vi "Optionen_2_Text.vi"(8 "error in (no error)":errorcluster caption="Fehler (Eingang, kein Fehler)", 9 "Abschnitt":string, 10 "Wartungsintervall:":sgl, 11 "Optionen":T1) -> (0 "error out":errorcluster caption="Fehler (Ausgang)", 3 "Array":string[](array[string]))   [LabVIEW 2020, in "System Einstellungen V2.lvlib"]
uses:
  System Einstellungen V2.lvlib
  Optionen.ctl
  <vilib>/Utility/Data Type/NI_Data Type.lvlib
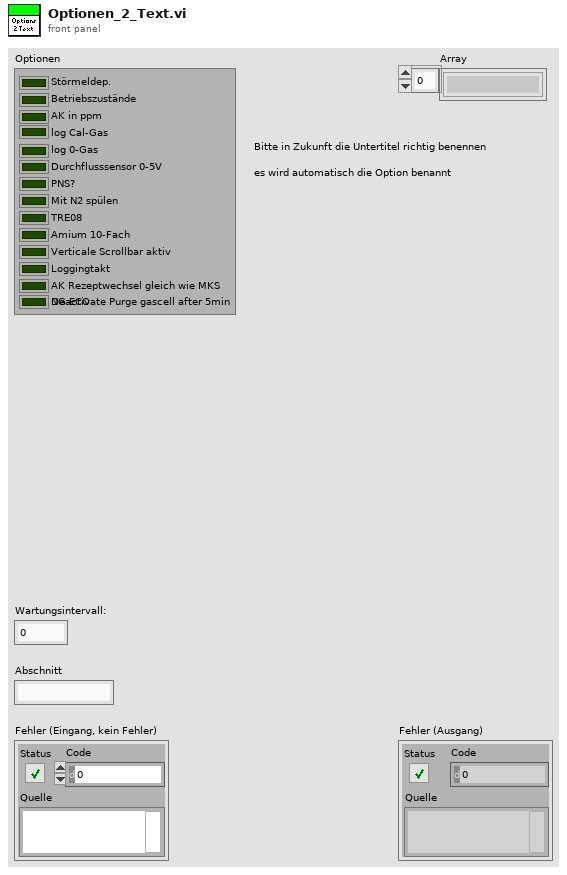
[diagram p1: front panel]
types:
  T1 = typedef "System Einstellungen V2.lvlib/Optionen.ctl" = cluster{"Störmeldep.":bool, "Betriebszustände":bool, "AK in ppm":bool, "log Cal-Gas":bool, "log 0-Gas":bool, "Durchflusssensor 0-5V":bool, "PNS?":bool, "Mit N2 spülen":bool, "TRE08":bool, "Amium 10-Fach":bool, "Verticale Scrollbar aktiv":bool, "Loggingtakt":bool, "AK Rezeptwechsel gleich wie MKS":bool, "NG ECO":bool}
  T2 = typedef "NI_Data Type.lvlib/Data Type.ctl" = enum8{"Invalid Type", "Void", "I8", "I16", "I32", "I64", "U8", "U16", "U32", "U64", "Single Float", "Double Float", "Extended Float", "Single Complex", "Double Complex", "Extended Complex", "Enum U8", "Enum U16", "Enum U32", "Enum U64", "Single Float With Unit", "Double Float With Unit", "Extended Float With Unit", "Single Complex with Unit", "Double Complex with Unit", "Extended Complex with Unit", "Boolean", "String", "Path", "Picture", "Tag", "Array", "Cluster", "Variant", "LV Variant", "Waveform", "Timestamp", "Digital Waveform", "Digital Data", "ExpressData", "Refnum", "External Data", "VI", "Poly VI", "LabVIEW Class Instance", "Fixed Point", "Set Collection", "Map Collection"}
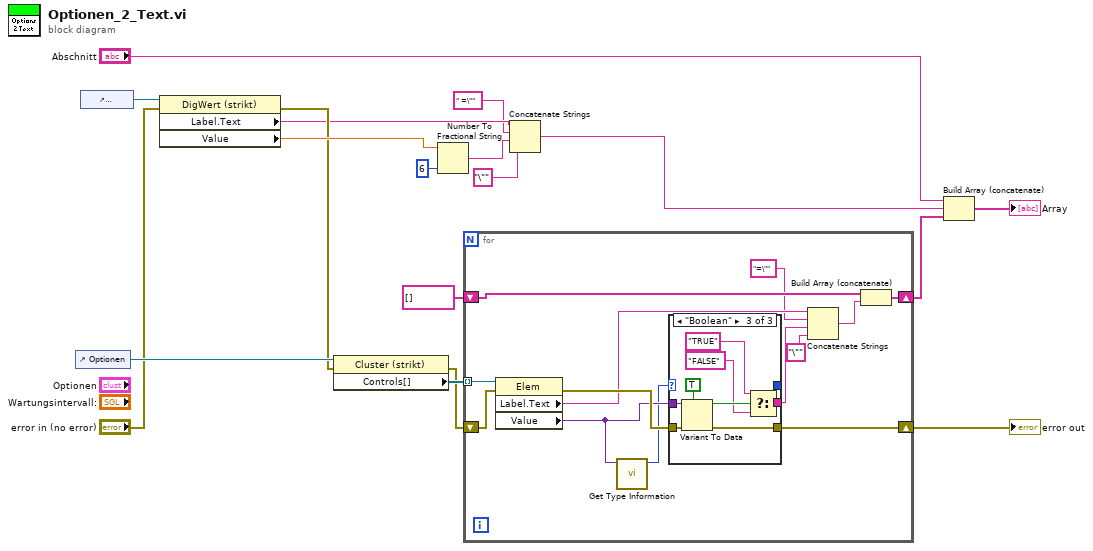
[diagram p0: block diagram]
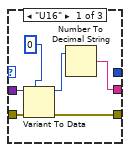
[diagram p2: hidden frame]
diagram:
  n1 = control-ref of="Optionen"() -> (w18:refnum<vi>)
  n2 = control-ref of="Wartungsintervall:"() -> (w12:refnum<vi>)
  n3 = property class="DigWert (strikt)"(reference=w12, error in="error in (no error)") -> (error out=w8:errorcluster, "Label.Text"=w4:string, "Value"=w11:sgl)  [unwired: 1 out]
  n4 = property class="Cluster (strikt)"(reference=w18, error in=w8) -> (error out=w16:errorcluster, "Controls[]"=w17:refnum<vi>[])  [unwired: 1 out]
  n5 = Number To Fractional String(number=w11, precision (6)=i16 6 ("Genauigkeit (6)")) -> (F-format string=w2:string)  [unwired: 2 in]
  n6 = for {
    tunnel: w17 -> [w28] mode=indexing
    shift-right: [w30] -> w15
    shift-left: w16 -> [w29]
    shift-right: [w26] -> w13
    shift-left: string[] [] -> [w25]
    n7 = property class="Elem"(reference=w28, error in=w29) -> (error out=w31:errorcluster, "Label.Text"=w24:string, "Value"=w20:variant)  [unwired: 1 out]
    n8 = call <vilib>:"Get Type Information.vi"("variant"=w20) -> ("type"=w19:T2)  [unwired: 6 in, 4 out]
    n9 = case shown="\"Boolean\"" w19 {
      selector: w19 -> [_ w38 _]
      tunnel: w31 -> [w36 w39 w45]
      tunnel: [w35 w39 w44] -> w30
      tunnel: [w32 _ w41] -> w22
      tunnel: w20 -> [w37 _ w40]
      tunnel: [_ w38 _] -> _
      frame "U16" {
        n10 = Variant To Data(error in=w36, type=u16 0, Variant=w37) -> (data=w33:u16, error out=w35:errorcluster)
        n11 = Number To Decimal String(number=w33) -> (decimal integer string=w32:string)  [unwired: 1 in]
      }
      frame "Invalid Type", Default {
      }
      frame "Boolean" {
        n12 = Variant To Data(error in=w45, type=TRUE, Variant=w40) -> (data=w46:bool, error out=w44:errorcluster)
        n13 = Select(t="TRUE", s=w46, f="FALSE") -> (s? t:f=w41:string)
      }
    }
    n14 = Concatenate Strings(w24, "=\"", w22, "\"") -> (w27:string)
    n15 = Build Array (concatenate)(w25, w27) -> (w26:string[])
  }
  "error out" <- w15
  n16 = Concatenate Strings(w4, " =\"", w2, "\"") -> (w6:string)
  n17 = Build Array (concatenate)("Abschnitt", w6, w13) -> (→"Array":string[])
